vi "5.2 1D-Cluster to CSM API String.vi"() -> ()   [LabVIEW 2017]
uses:
  9f1c8977-aa41-4596-a18a-6dba2ebc59d2.vi
  0333efe5-f0fb-4901-b6dd-db031cec30c6.vi
  addons/API-String-Arugments-Support/_Support/Data To API String Arguments.vi
  addons/API-String-Arugments-Support/_Support/Convert API String Arguments to Data(variant).vi
panel:
  out "Flattened String":string
  in  "Array":cluster{"String":string, "BoolArray":bool[]}[](array[cluster])=[{"String"="abc", "BoolArray"=[TRUE, FALSE, TRUE, FALSE]}, {"String"="def", "BoolArray"=[FALSE, TRUE, FALSE, TRUE]}, {"String"="xyz", "BoolArray"=[TRUE, TRUE, FALSE, FALSE]}]
  out "Array":cluster{"String":string, "BoolArray":bool[]}[](array[cluster])=[{"String"="abc", "BoolArray"=[TRUE, FALSE, TRUE, FALSE]}, {"String"="def", "BoolArray"=[FALSE, TRUE, FALSE, TRUE]}, {"String"="xyz", "BoolArray"=[TRUE, TRUE, FALSE, FALSE]}]
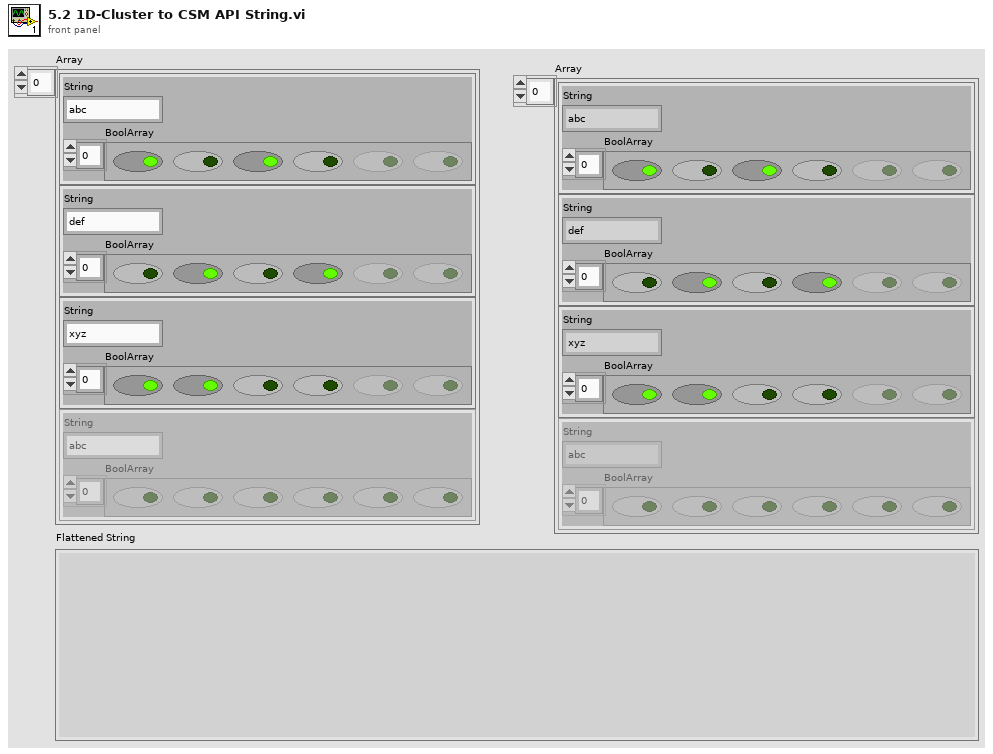
[diagram p1: front panel]
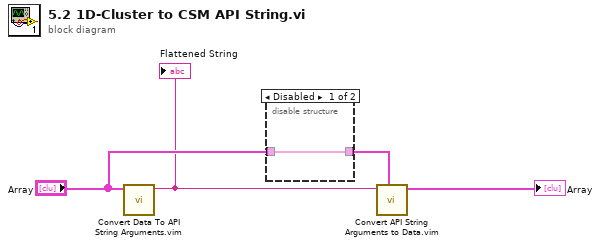
[diagram p0: block diagram]
diagram:
  n1 = call "Convert Data To API String Arguments.vim"("data"="Array") -> ("String"=w1:string)  [unwired: 7 in, 1 out]
  "Flattened String" <- w1
  n2 = disable-structure "Diagram Disable Structure" shown="Disabled" {
    disable-tunnel: "Array" -> [w5 _]
    disable-tunnel: [w5 _] -> w3
    frame Disabled {
    }
    frame Enabled {
    }
  }
  n3 = call "Convert API String Arguments to Data.vim"("Type"=w3, "String"=w1) -> ("Data"=→"Array":cluster{"String":string, "BoolArray":bool[]}[])  [unwired: 6 in, 1 out]
